vi "LightFieldInit.vi"(0 "LightField Automation in":refnum<class "LightField Automation.lvclass">, 2 "MODE":u16(ring) items=["Normal", "DIF"], 3 "BIN":u16(ring) items=["1x1", "2x2", "4x4"], 5 "error in":errorcluster, 6 "Initial Gate Delay (us)":dbl, 7 "Initial Gate Width (us)":dbl, 8 "Number of Frames":i32=500 min=0 step=1, 9 "File Path":refnum<file>, 10 "On CCD Accumulations":i32=3 min=0 step=1, 12 "Second Gate Delay (us)":dbl, 13 "Second Gate Width (us)":dbl) -> (14 "LightField Automation out":refnum<class "LightField Automation.lvclass">, 19 "error out":errorcluster)   [LabVIEW 2018]
uses:
  <userlib>/LightField Add-in and Automation SDK/Samples/LabVIEW Automation/lightfield-automation-labview/LightField Automation.lvclass
  C:/Program Files/Princeton Instruments/LightField/PrincetonInstruments.LightFieldAddInSupportServices.dll
  Program Files/Princeton Instruments/LightField/PrincetonInstruments.LightFieldAddInSupportServices.dll
  C:/Program Files/Princeton Instruments/LightField/AddInViews/PrincetonInstruments.LightFieldViewV3.dll
  Program Files/Princeton Instruments/LightField/AddInViews/PrincetonInstruments.LightFieldViewV3.dll
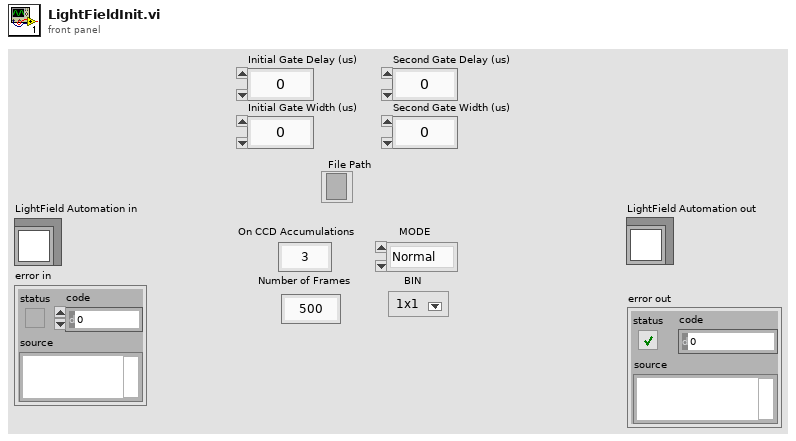
[diagram p1: front panel]
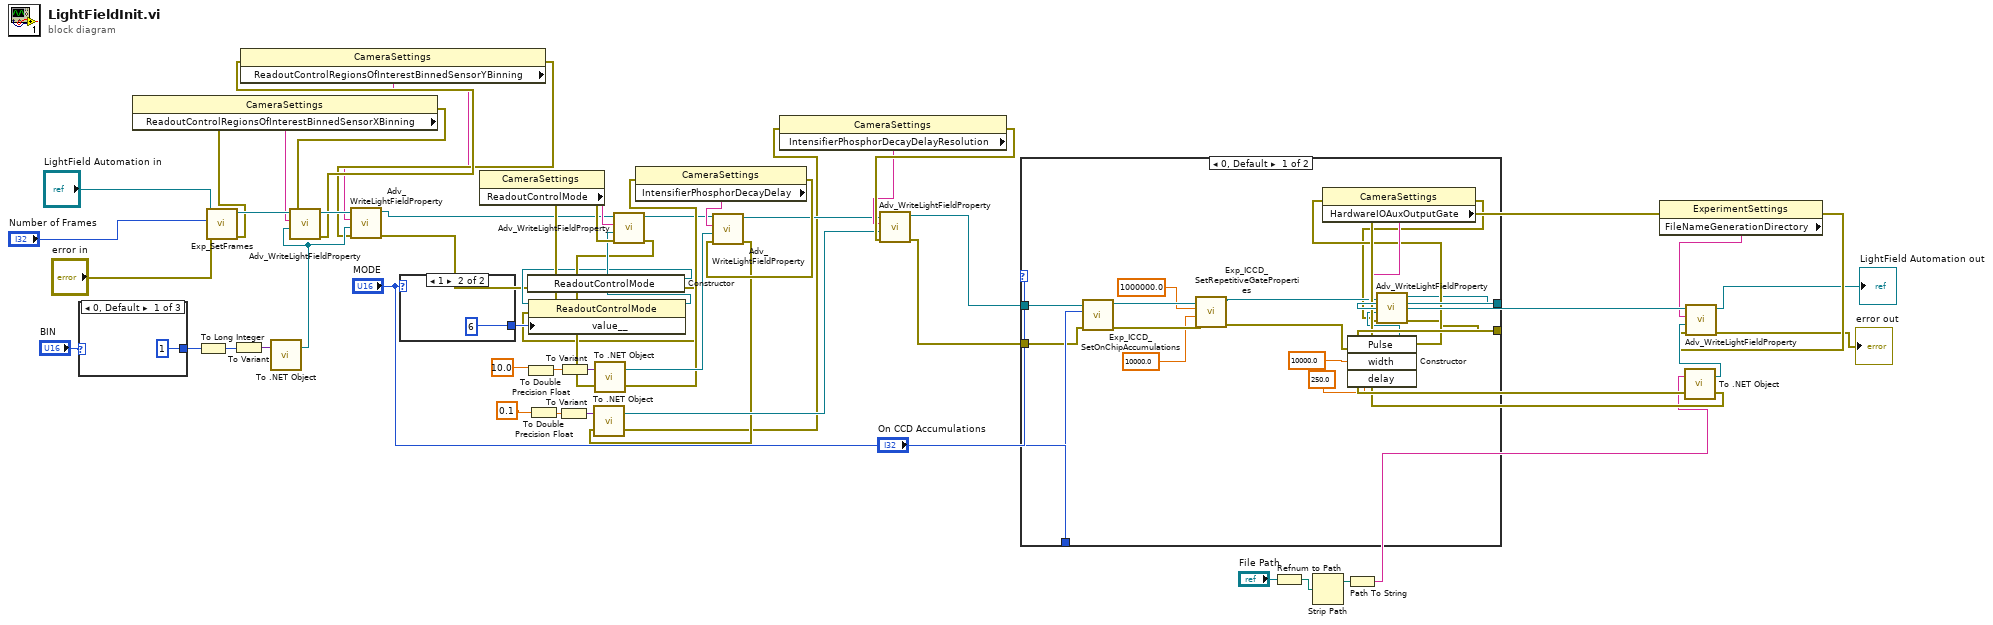
[diagram p0: block diagram]
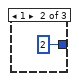
[diagram p2: hidden frame]
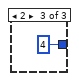
[diagram p3: hidden frame]
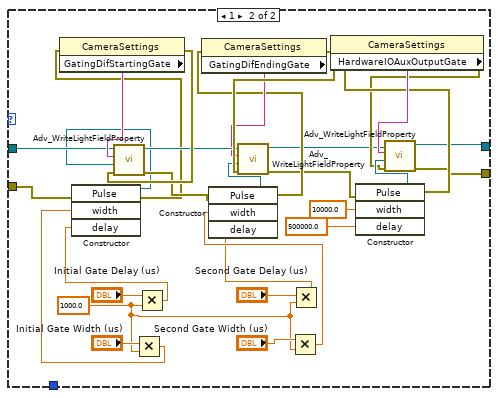
[diagram p4: hidden frame]
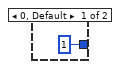
[diagram p5: hidden frame]
diagram:
  n1 = case shown="0, Default" "BIN" {
    tunnel: [1 2 4] -> w27
    frame 0, Default {
    }
    frame 1 {
    }
    frame 2 {
    }
  }
  n2 = To Long Integer(number=w27) -> (32bit integer=w26:i32)
  n3 = call <userlib>:"Exp_SetFrames.vi"("error in (no error)"="error in", "Number of Frames"="Number of Frames", "LightField Automation in"="LightField Automation in") -> ("error out"=w38:errorcluster, "LightField Automation out"=w56:refnum<class "LightField Automation.lvclass">)  [unwired: 7 in]
  n4 = property class="CameraSettings"(error in=w38) -> (error out=w37:errorcluster, "ReadoutControlRegionsOfInterestBinnedSensorXBinning"=w36:string)  [unwired: 1 in, 1 out]
  n5 = To Variant(anything=w26) -> (Variant=w35:variant)
  n6 = call <vilib>:"To .NET Object.vi"("anything"=w35) -> (".NET object"=w34:refnum<k24>)  [unwired: 1 in, 1 out]
  n7 = call <userlib>:"Adv_WriteLightFieldProperty.vi"("error in (no error)"=w37, "value"=w34, "setting"=w36, "LightField Automation in"=w56) -> ("error out"=w33:errorcluster, "LightField Automation out"=w41:refnum<class "LightField Automation.lvclass">)  [unwired: 6 in]
  n8 = property class="CameraSettings"(error in=w33) -> (error out=w32:errorcluster, "ReadoutControlRegionsOfInterestBinnedSensorYBinning"=w31:string)  [unwired: 1 in, 1 out]
  n9 = call <userlib>:"Adv_WriteLightFieldProperty.vi"("error in (no error)"=w32, "value"=w34, "setting"=w31, "LightField Automation in"=w41) -> ("error out"=w29:errorcluster, "LightField Automation out"=w40:refnum<class "LightField Automation.lvclass">)  [unwired: 6 in]
  n10 = case shown="1" "MODE" {
    tunnel: [1 ("value__") 6 ("value__")] -> w53
    frame 0, Default {
    }
    frame 1 {
    }
  }
  n11 = To Double Precision Float(number=10.0) -> (double precision float=w25:dbl)
  n12 = constructor class="ReadoutControlMode"(error in=w29) -> (reference out=w30:refnum<k24>, error out=w28:errorcluster)  [unwired: 2 in, 1 out]
  n13 = property class="ReadoutControlMode"(reference=w30, error in=w28, "value__"=w53) -> (reference out=w52:refnum<k24>, error out=w51:errorcluster)
  n14 = property class="CameraSettings"(error in=w51) -> (error out=w54:errorcluster, "ReadoutControlMode"=w55:string)  [unwired: 1 in, 1 out]
  n15 = To Double Precision Float(number=0.1) -> (double precision float=w10:dbl)
  n16 = To Variant(anything=w10) -> (Variant=w11:variant)
  n17 = To Variant(anything=w25) -> (Variant=w49:variant)
  n18 = call <userlib>:"Adv_WriteLightFieldProperty.vi"("error in (no error)"=w54, "value"=w52, "setting"=w55, "LightField Automation in"=w40) -> ("error out"=w48:errorcluster, "LightField Automation out"=w44:refnum<class "LightField Automation.lvclass">)  [unwired: 6 in]
  n19 = call <vilib>:"To .NET Object.vi"("error in (no error)"=w48, "anything"=w49) -> ("error out"=w46:errorcluster, ".NET object"=w47:refnum<k24>)
  n20 = property class="CameraSettings"(error in=w46) -> (error out=w45:errorcluster, "IntensifierPhosphorDecayDelay"=w50:string)  [unwired: 1 in, 1 out]
  n21 = call <userlib>:"Adv_WriteLightFieldProperty.vi"("error in (no error)"=w45, "value"=w47, "setting"=w50, "LightField Automation in"=w44) -> ("error out"=w6:errorcluster, "LightField Automation out"=w7:refnum<class "LightField Automation.lvclass">)  [unwired: 6 in]
  n22 = call <vilib>:"To .NET Object.vi"("error in (no error)"=w6, "anything"=w11) -> ("error out"=w5:errorcluster, ".NET object"=w9:refnum<k24>)
  n23 = property class="CameraSettings"(error in=w5) -> (error out=w12:errorcluster, "IntensifierPhosphorDecayDelayResolution"=w8:string)  [unwired: 1 in, 1 out]
  n24 = call <userlib>:"Adv_WriteLightFieldProperty.vi"("error in (no error)"=w12, "value"=w9, "setting"=w8, "LightField Automation in"=w7) -> ("error out"=w4:errorcluster, "LightField Automation out"=w3:refnum<class "LightField Automation.lvclass">)  [unwired: 6 in]
  n25 = case shown="0, Default" "MODE" {
    tunnel: "On CCD Accumulations" -> [w81 _]
    tunnel: w4 -> [w80 w102]
    tunnel: w3 -> [w79 w111]
    tunnel: [w69 w93] -> w24
    tunnel: [w68 w92] -> w23
    frame 0, Default {
      n26 = call <userlib>:"Exp_ICCD_SetOnChipAccumulations.vi"("error in (no error)"=w80, "On Chip Accumulations"=w81, "LightField Automation in"=w79) -> ("error out"=w78:errorcluster, "LightField Automation out"=w77:refnum<class "LightField Automation.lvclass">)  [unwired: 7 in]
      n27 = call <userlib>:"Exp_ICCD_SetRepetitiveGateProperties.vi"("error in (no error)"=w78, "Repetitive Gate Width (ns)"=10000.0, "Repetitive Gate Delay (ns)"=1000000.0, "LightField Automation in"=w77) -> ("error out"=w70:errorcluster, "LightField Automation out"=w71:refnum<class "LightField Automation.lvclass">)  [unwired: 6 in]
      n28 = constructor class="Pulse"(error in=w70, "width"=10000.0 ("delay"), "delay"=250.0 ("width")) -> (reference out=w72:refnum<k24>, error out=w73:errorcluster)  [unwired: 2 in, 3 out]
      n29 = property class="CameraSettings"(error in=w73) -> (error out=w67:errorcluster, "HardwareIOAuxOutputGate"=w74:string)  [unwired: 1 in, 1 out]
      n30 = call <userlib>:"Adv_WriteLightFieldProperty.vi"("error in (no error)"=w67, "value"=w72, "setting"=w74, "LightField Automation in"=w71) -> ("error out"=w69:errorcluster, "LightField Automation out"=w68:refnum<class "LightField Automation.lvclass">)  [unwired: 6 in]
    }
    frame 1 {
      w86 = 1000.0 ("y")
      n31 = Multiply(x="Initial Gate Width (us)", y=w86) -> (x*y=w82:dbl)
      n32 = Multiply(x="Initial Gate Delay (us)", y=w86) -> (x*y=w83:dbl)
      n33 = constructor class="Pulse"(error in=w102, "width"=w82, "delay"=w83) -> (reference out=w103:refnum<k24>, error out=w101:errorcluster)  [unwired: 2 in, 3 out]
      n34 = property class="CameraSettings"(error in=w101) -> (error out=w110:errorcluster, "GatingDifStartingGate"=w112:string)  [unwired: 1 in, 1 out]
      n35 = call <userlib>:"Adv_WriteLightFieldProperty.vi"("error in (no error)"=w110, "value"=w103, "setting"=w112, "LightField Automation in"=w111) -> ("error out"=w106:errorcluster, "LightField Automation out"=w108:refnum<class "LightField Automation.lvclass">)  [unwired: 6 in]
      n36 = Multiply(x="Second Gate Width (us)", y=w86) -> (x*y=w85:dbl)
      n37 = Multiply(x="Second Gate Delay (us)", y=w86) -> (x*y=w84:dbl)
      n38 = constructor class="Pulse"(error in=w106, "width"=w85, "delay"=w84) -> (reference out=w104:refnum<k24>, error out=w105:errorcluster)  [unwired: 2 in, 3 out]
      n39 = property class="CameraSettings"(error in=w105) -> (error out=w109:errorcluster, "GatingDifEndingGate"=w107:string)  [unwired: 1 in, 1 out]
      n40 = call <userlib>:"Adv_WriteLightFieldProperty.vi"("error in (no error)"=w109, "value"=w104, "setting"=w107, "LightField Automation in"=w108) -> ("error out"=w94:errorcluster, "LightField Automation out"=w91:refnum<class "LightField Automation.lvclass">)  [unwired: 6 in]
      n41 = constructor class="Pulse"(error in=w94, "width"=10000.0, "delay"=500000.0) -> (reference out=w98:refnum<k24>, error out=w99:errorcluster)  [unwired: 2 in, 3 out]
      n42 = property class="CameraSettings"(error in=w99) -> (error out=w95:errorcluster, "HardwareIOAuxOutputGate"=w100:string)  [unwired: 1 in, 1 out]
      n43 = call <userlib>:"Adv_WriteLightFieldProperty.vi"("error in (no error)"=w95, "value"=w98, "setting"=w100, "LightField Automation in"=w91) -> ("error out"=w93:errorcluster, "LightField Automation out"=w92:refnum<class "LightField Automation.lvclass">)  [unwired: 6 in]
    }
  }
  n44 = Refnum to Path(1:"File Path") -> (0:w21:path)
  n45 = Strip Path(path=w21) -> (stripped path=w20:path)  [unwired: 1 out]
  n46 = Path To String(path=w20) -> (string=w15:string)
  n47 = call <vilib>:"To .NET Object.vi"("error in (no error)"=w24, "anything"=w15) -> ("error out"=w16:errorcluster, ".NET object"=w18:refnum<k24>)
  n48 = property class="ExperimentSettings"(error in=w16) -> (error out=w17:errorcluster, "FileNameGenerationDirectory"=w19:string)  [unwired: 1 in, 1 out]
  n49 = call <userlib>:"Adv_WriteLightFieldProperty.vi"("error in (no error)"=w17, "value"=w18, "setting"=w19, "LightField Automation in"=w23) -> ("error out"=→"error out":errorcluster, "LightField Automation out"=→"LightField Automation out":refnum<class "LightField Automation.lvclass">)  [unwired: 6 in]
